vi "Write Overall Test Result.vi"(7 "Data Repo in":refnum<class "Data Repo.lvclass">, 10 "Tests Passed":bool[](array[boolean]), 11 "Test Class in":refnum<class "Test Class.lvclass">) -> ()   [LabVIEW 2017, in "Test Class.lvclass"]
uses:
  Test Class.lvclass
  <vilib>/TSS/ACRObat Test Framework/Classes/Data/Data Repo/Class/Data Repo.lvclass
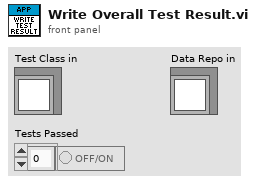
[diagram p1: front panel]
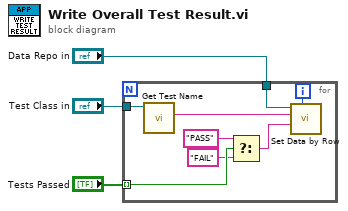
[diagram p0: block diagram]
diagram:
  n1 = for {
    tunnel: "Tests Passed" -> [w7] mode=indexing
    tunnel: "Test Class in" -> [w10]
    tunnel: "Data Repo in" -> [w9]
    i -> [w11]
    n2 = call "Get Test Name.vi"("Test Class in"=w10) -> ("Test Name"=w8:string)  [unwired: 9 in, 1 out]
    n3 = Select(t="PASS", s=w7, f="FAIL") -> (s? t:f=w4:string)
    n4 = call <vilib>:"Set Data by Row.vi"("Row"=w11, "Value"=w4, "Header"=w8, "Acrobat Template in"=w9) -> ()  [unwired: 6 in, 2 out]
  }
